vi "calcStiffness.vi"(8 "error in (no error)":errorcluster, 11 "Model in":refnum<class "Model.lvclass">) -> (0 "error out":errorcluster, 3 "Model out":refnum<class "Model.lvclass">)   [LabVIEW 2013, in "Model.lvclass"]
uses:
  Model.lvclass
  Typedefs/StiffnessData.ctl
  Model.lvclass/Model.ctl
  UserEvents/UserEvents.lvclass/UserEvents.ctl
  ApplicationElements/DistanceGauge/DistanceGauge.lvclass/DistanceGauge.ctl
  ApplicationElements/StiffnessMonitor/StiffnessMonitor.lvclass/StiffnessMonitor.ctl
  ApplicationElements/Encoder/Encoder.lvclass/Encoder.ctl
  ApplicationElements/ForceSensor/ForceSensor.lvclass/ForceSensor.ctl
  ApplicationElements/Log/StiffnessLog/StiffnessLog.lvclass/StiffnessLog.ctl
  ApplicationElements/StiffnessMonitor/StiffnessMonitor.lvclass
  Typedefs/M2AADTTypedefs.lvlib
  UserEvents/UserEvents.lvclass
  ApplicationElements/DistanceGauge/DistanceGauge.lvclass
  ApplicationElements/Encoder/Encoder.lvclass
  ApplicationElements/ForceSensor/ForceSensor.lvclass
  ApplicationElements/Log/StiffnessLog/StiffnessLog.lvclass
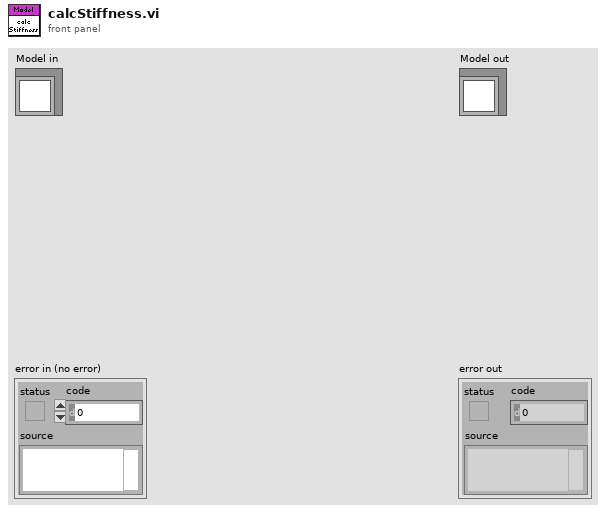
[diagram p1: front panel]
types:
  T1 = typedef "M2AADTTypedefs.lvlib/StiffnessData.ctl" = cluster{"Constrained Displacement":dbl[unit], "Stiffness":dbl[unit]}
  T2 = typedef "M2AADTTypedefs.lvlib/PubDataEvents.ctl" = cluster{"State":refnum<user-event>, "ErrorCode":refnum<user-event>, "OutputData":refnum<user-event>, "InputData":refnum<user-event>, "ControllerData":refnum<user-event>, "TestStatus":refnum<user-event>, "LogPath":refnum<user-event>, "StiffnessData":refnum<user-event>}
  T3 = typedef "M2AADTTypedefs.lvlib/Distance Data.ctl" = cluster{"Distance Measured 1":dbl[unit], "Distance Measured 2":dbl[unit]}
  T4 = typedef "M2AADTTypedefs.lvlib/ForceDemand.ctl" = dbl[unit]
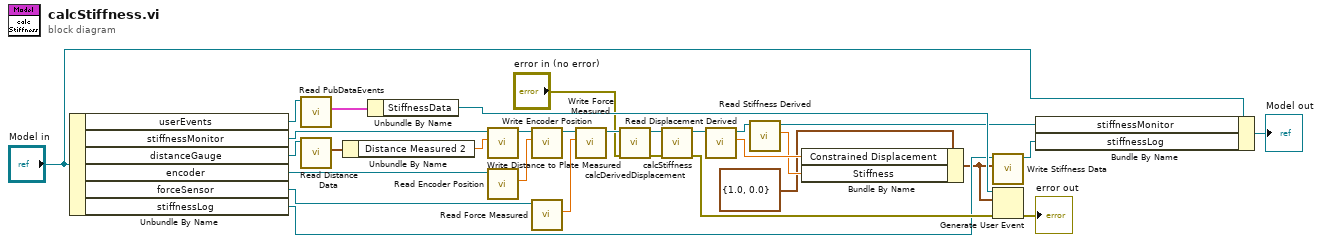
[diagram p0: block diagram]
diagram:
  n1 = Unbundle By Name("Model in") -> ("userEvents"=w21:refnum<class "UserEvents.lvclass">, "stiffnessMonitor"=w11:refnum<class "StiffnessMonitor.lvclass">, "distanceGauge"=w17:refnum<class "DistanceGauge.lvclass">, "encoder"=w15:refnum<class "Encoder.lvclass">, "forceSensor"=w13:refnum<class "ForceSensor.lvclass">, "stiffnessLog"=w6:refnum<class "StiffnessLog.lvclass">)
  n2 = call "Read PubDataEvents.vi"("UserEvents in"=w21) -> ("PubDataEvents"=w23:T2)  [unwired: 9 in, 1 out]
  n3 = call "Read Distance Data.vi"("DistanceGauge in"=w17) -> ("Distance Data"=w18:T3)  [unwired: 9 in, 1 out]
  n4 = Unbundle By Name(w18) -> ("Distance Measured 2"=w19:dbl[unit])
  n5 = Unbundle By Name(w23) -> ("StiffnessData"=w22:refnum<user-event>)
  n6 = call "Write Distance to Plate Measured.vi"("Distance to Plate Measured"=w19, "StiffnessMonitor in"=w11) -> ("StiffnessMonitor out"=w20:refnum<class "StiffnessMonitor.lvclass">)  [unwired: 9 in]
  n7 = call "Read Encoder Position.vi"("Encoder in"=w15) -> ("Encoder Position"=w16:dbl[unit])  [unwired: 9 in, 1 out]
  n8 = call "Write Encoder Position.vi"("Encoder Position"=w16, "StiffnessMonitor in"=w20) -> ("StiffnessMonitor out"=w14:refnum<class "StiffnessMonitor.lvclass">)  [unwired: 9 in]
  n9 = call "Read Force Measured.vi"("ForceSensor in"=w13) -> ("Force Demand"=w12:T4)  [unwired: 9 in, 1 out]
  n10 = call "Write Force Measured.vi"("Force Measured"=w12, "StiffnessMonitor in"=w14) -> ("StiffnessMonitor out"=w30:refnum<class "StiffnessMonitor.lvclass">)  [unwired: 9 in]
  n11 = call "calcDerivedDisplacement.vi"("error in (no error)"="error in (no error)", "StiffnessMonitor in"=w30) -> ("error out"=w9:errorcluster, "StiffnessMonitor out"=w29:refnum<class "StiffnessMonitor.lvclass">)  [unwired: 8 in]
  n12 = call "calcStiffness.vi"("error in (no error)"=w9, "StiffnessMonitor in"=w29) -> ("error out"=w8:errorcluster, "StiffnessMonitor out"=w28:refnum<class "StiffnessMonitor.lvclass">)  [unwired: 8 in]
  n13 = call "Read Displacement Derived.vi"("StiffnessMonitor in"=w28) -> ("Displacement Derived"=w26:dbl[unit], "StiffnessMonitor out"=w27:refnum<class "StiffnessMonitor.lvclass">)  [unwired: 9 in]
  n14 = call "Read Stiffness Derived.vi"("StiffnessMonitor in"=w27) -> ("Stiffness Derived"=w25:dbl[unit], "StiffnessMonitor out"=w2:refnum<class "StiffnessMonitor.lvclass">)  [unwired: 9 in]
  n15 = Bundle By Name(cluster=T1 {"Constrained Displacement"=1.0, "Stiffness"=0.0} ("event data"), "Constrained Displacement"=w26, "Stiffness"=w25) -> (w1:T1)
  n16 = call "Write Stiffness Data.vi"("Stiffness Data"=w1, "StiffnessLog in"=w6) -> ("StiffnessLog out"=w3:refnum<class "StiffnessLog.lvclass">)  [unwired: 9 in]
  n17 = Generate User Event(user event=w22, event data cluster=w1, error in=w8) -> (error out=→"error out":errorcluster)  [unwired: 1 in, 1 out]
  n18 = Bundle By Name(cluster="Model in", "stiffnessMonitor"=w2, "stiffnessLog"=w3) -> (→"Model out":refnum<class "Model.lvclass">)
